vi "runServer.vi"(8 "error in (no error)":errorcluster, 11 "TcpServer in":refnum<class "TcpServer.lvclass">) -> (0 "error out (no error)":errorcluster, 3 "TcpServer out":refnum<class "TcpServer.lvclass">)   [LabVIEW 2018, in "TcpServer.lvclass"]
doc: "Run the TCP Server."
uses:
  TcpServer.lvclass
  TcpServer.lvclass/TcpServer.ctl
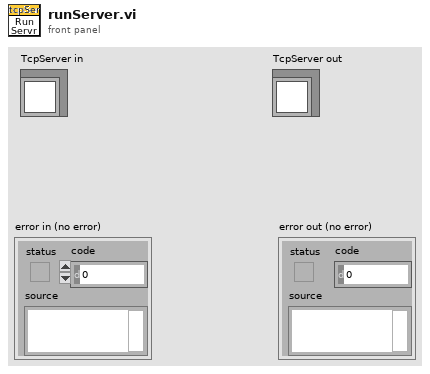
[diagram p1: front panel]
types:
  T1 = typedef "TcpServer.lvclass/userEventsTypeDef.ctl" = cluster{"TcpServer":refnum<user-event>, "Cmd":refnum<user-event>, "CmdStatus":refnum<user-event>, "Event":refnum<user-event>}
  T2 = enum16{"Standard", "Buffered", "CRLF", "Immediate"}
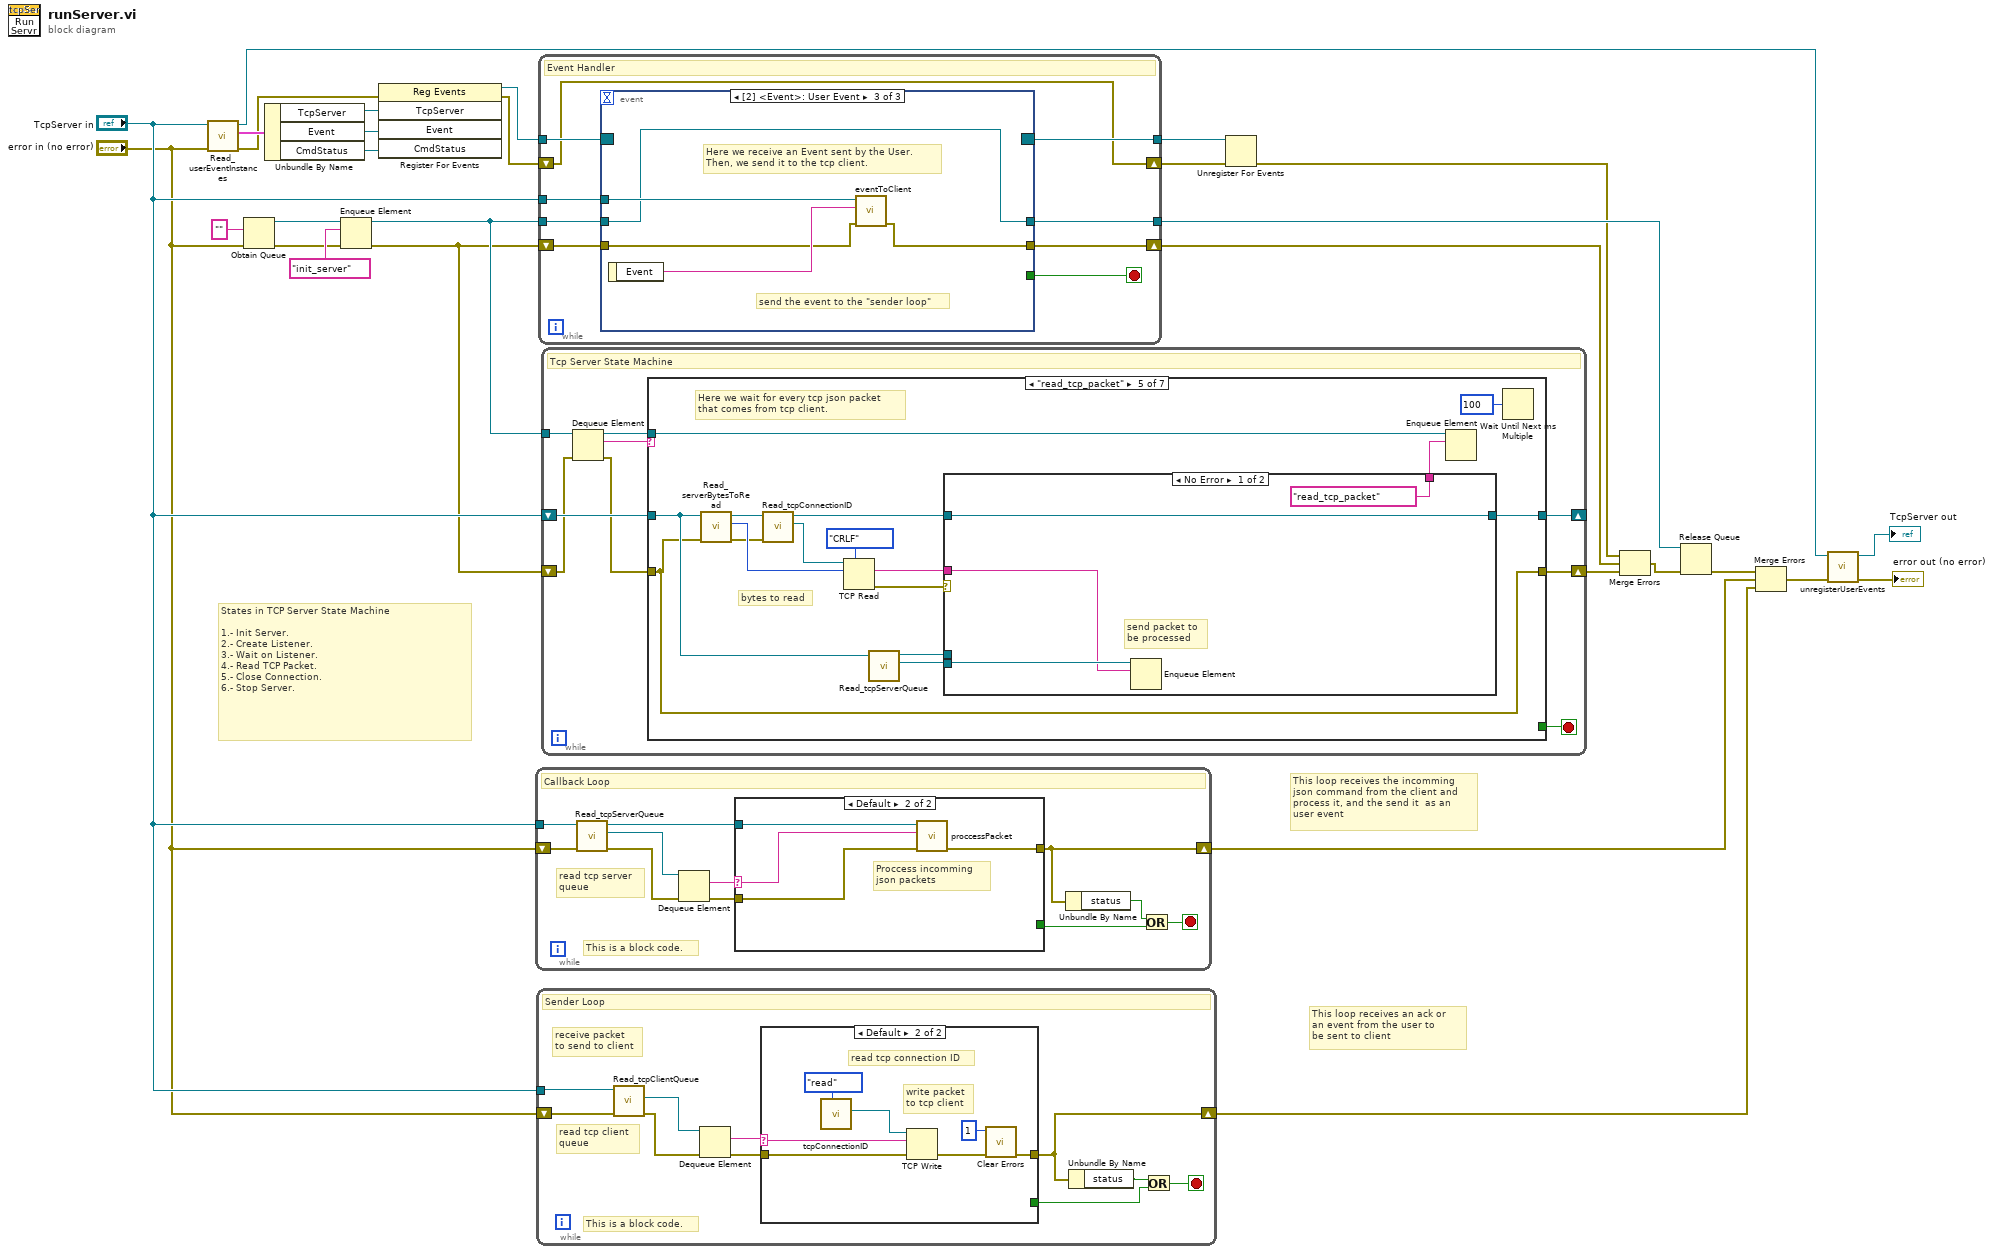
[diagram p0: block diagram]
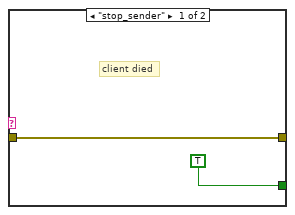
[diagram p2: hidden frame]
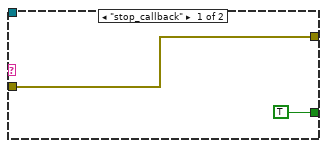
[diagram p3: hidden frame]
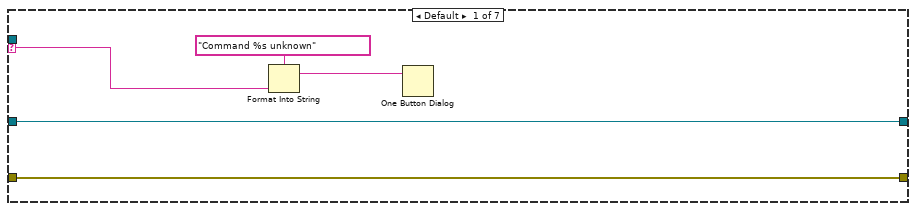
[diagram p4: hidden frame]
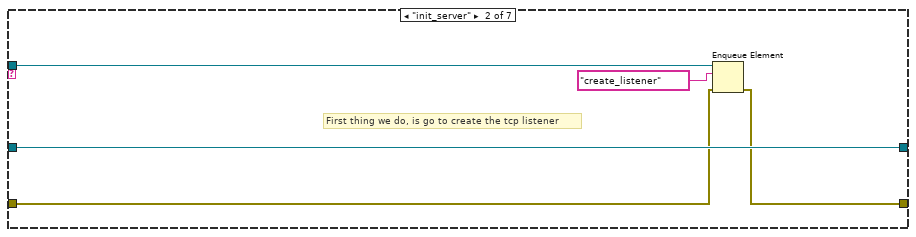
[diagram p5: hidden frame]
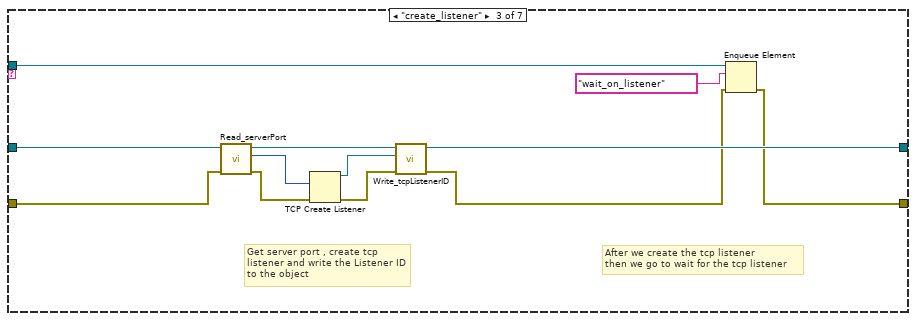
[diagram p6: hidden frame]
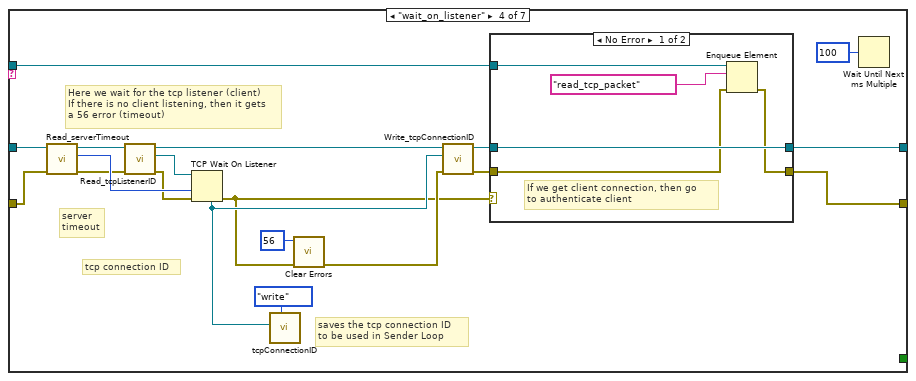
[diagram p7: hidden frame]
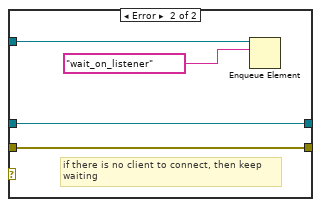
[diagram p8: hidden frame]
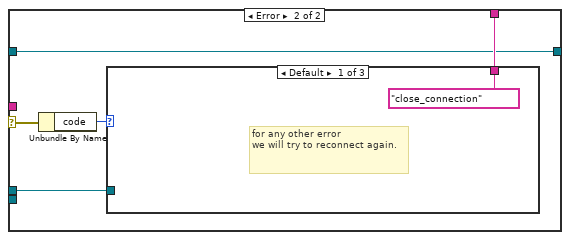
[diagram p9: hidden frame]
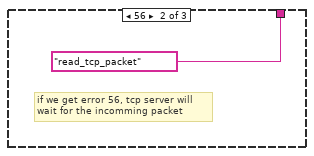
[diagram p10: hidden frame]
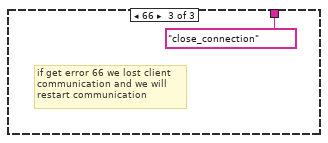
[diagram p11: hidden frame]
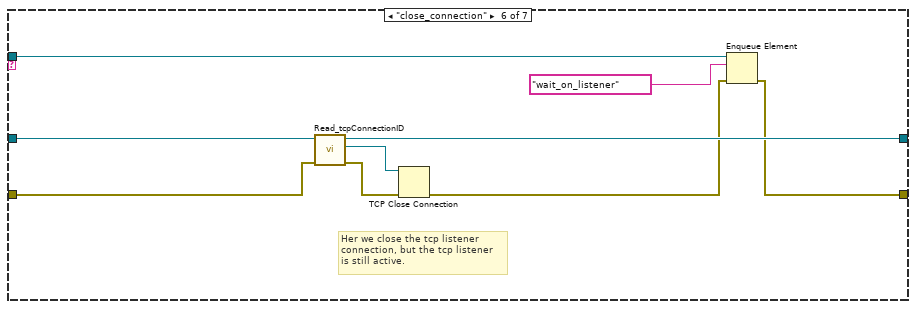
[diagram p12: hidden frame]
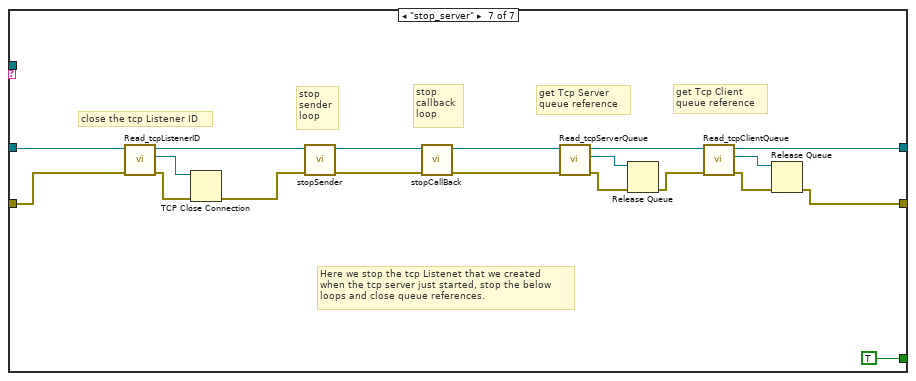
[diagram p13: hidden frame]
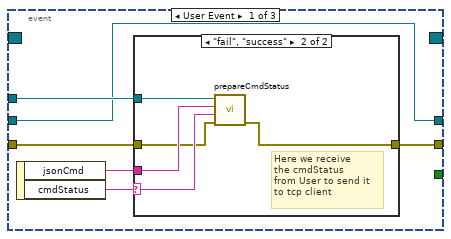
[diagram p14: hidden frame]
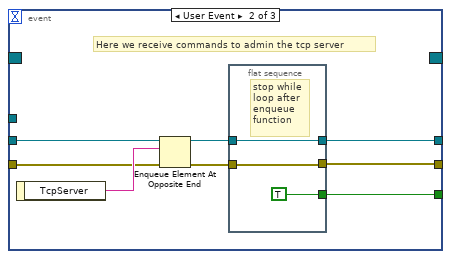
[diagram p16: hidden frame]
diagram:
  # "States in TCP Server State Machine\n\n1.- Init Server.\n2.- Create Listener.\n3.- Wait on Listener.\n4.- Read TCP Packet.\n5.- Close Connection.\n6.- Stop Server."
  # "This loop receives an ack or\nan event from the user to\nbe sent to client"
  # "This loop receives the incomming\njson command from the client and\nprocess it, and the send it  as an \nuser event"
  n1 = call "Read_userEventInstances.vi"("error in (no error)"="error in (no error)", "tcpServer in"="TcpServer in") -> ("error out"=w6:errorcluster, "UserEvents"=w27:T1, "tcpServer out"=w10:refnum<class "TcpServer.lvclass">)  [unwired: 7 in]
  n2 = Obtain Queue(element data type="", error in (no error)="error in (no error)") -> (queue out=w28:refnum<queue>, error out=w12:errorcluster)  [unwired: 3 in, 1 out]
  n3 = Unbundle By Name(w27) -> ("TcpServer"=w26:refnum<user-event>, "Event"=w21:refnum<user-event>, "CmdStatus"=w16:refnum<user-event>)
  n4 = Enqueue Element(queue=w28, element="init_server", error in (no error)=w12) -> (queue out=w24:refnum<queue>, error out=w7:errorcluster)  [unwired: 1 in, 1 out]
  n5 = register-events(error in=w6, w26, w21, w16) -> (reference out=w25:refnum<event-registration>, error out=w5:errorcluster)  [unwired: 1 in]
  n6 = while {
    tunnel: "TcpServer in" -> [w37]
    shift-right: [w31] -> w14
    shift-left: "error in (no error)" -> [w36]
    stop <- w33 stop-if-true
    # "This is a block code."
    # "read tcp server \nqueue"
    # "Callback Loop"
    n7 = call "Read_tcpServerQueue.vi"("error in (no error)"=w36, "tcpServer in"=w37) -> ("error out"=w35:errorcluster, "tcpServer queue"=w40:refnum<queue>, "tcpServer out"=w39:refnum<class "TcpServer.lvclass">)  [unwired: 7 in]
    n8 = Dequeue Element(queue=w40, error in (no error)=w35) -> (element=w38:string, error out=w34:errorcluster)  [unwired: 1 in, 2 out]
    n9 = case shown="Default" w38 {
      selector: w38 -> [_ w45]
      tunnel: w39 -> [_ w46]
      tunnel: [TRUE _] -> w32
      tunnel: w34 -> [w41 w44]
      tunnel: [w41 w43] -> w31
      frame "stop_callback" {
      }
      frame Default {
        # "Proccess incomming\njson packets"
        n10 = call "proccessPacket.vi"("error in (no error)"=w44, "tcp packet"=w45, "tcpServer in"=w46) -> ("error out"=w43:errorcluster)  [unwired: 7 in, 1 out]
      }
    }
    n11 = Unbundle By Name(w31) -> ("status"=w30:bool)
    n12 = Or(x=w30, y=w32) -> (x .or. y?=w33:bool)
  }
  n13 = while {
    tunnel: "TcpServer in" -> [w56]
    shift-right: [w47] -> w13
    shift-left: "error in (no error)" -> [w53]
    stop <- w52 stop-if-true
    # "This is a block code."
    # "receive packet\nto send to client"
    # "read tcp client \nqueue"
    # "Sender Loop"
    n14 = call "Read_tcpClientQueue.vi"("error in (no error)"=w53, "tcpServer in"=w56) -> ("error out"=w50:errorcluster, "tcpClient queue"=w54:refnum<queue>)  [unwired: 7 in, 1 out]
    n15 = Dequeue Element(queue=w54, error in (no error)=w50) -> (element=w55:string, error out=w49:errorcluster)  [unwired: 1 in, 2 out]
    n16 = case shown="Default" w55 {
      selector: w55 -> [_ w65]
      tunnel: [TRUE _] -> w51
      tunnel: w49 -> [w57 w59]
      tunnel: [w57 w60] -> w47
      frame "stop_sender" {
        # "client died"
      }
      frame Default {
        # "write packet\nto tcp client"
        # "read tcp connection ID"
        n17 = call "tcpConnectionID.vi"("function"=enum16{"read", "write"}."read") -> ("connection ID out"=w63:refnum<k5>)  [unwired: 10 in]
        n18 = TCP Write(connection ID=w63, data in=w65, error in (no error)=w59) -> (error out=w61:errorcluster)  [unwired: 1 in, 2 out]
        n19 = call <vilib>:"Clear Errors.vi"("error in (no error)"=w61, "specific error code to clear (0: all)"=1) -> ("error out"=w60:errorcluster)  [unwired: 4 in, 1 out]
      }
    }
    n20 = Unbundle By Name(w47) -> ("status"=w48:bool)
    n21 = Or(x=w48, y=w51) -> (x .or. y?=w52:bool)
  }
  n22 = while {
    tunnel: w24 -> [w74]
    tunnel: w25 -> [w73]
    tunnel: [w71] -> w22
    tunnel: "TcpServer in" -> [w70]
    tunnel: [w69] -> w8
    shift-right: [w66] -> w3
    shift-left: w5 -> [w66]
    shift-right: [w67] -> w1
    shift-left: w7 -> [w68]
    stop <- w72 stop-if-true
    # "Event Handler"
    n23 = event shown="[2] <Event>: User Event" {
      selector: w73 -> [_ _ _]
      dyn-events: [_ _ _] -> w69
      timeout: _ -> [_ _ _]
      tunnel: w74 -> [w75 w94 w100]
      tunnel: [_ w92 _] -> w72
      tunnel: [w75 w90 w100] -> w71
      tunnel: w70 -> [w78 _ w102]
      tunnel: w68 -> [w77 w89 w99]
      tunnel: [w76 w87 w98] -> w67
      event User Event {
        n24 = event-data() -> ("jsonCmd"=w79:string, "cmdStatus"=w80:string)  [unwired: 1 in]
        n25 = case shown="\"fail\", \"success\"" w80 {
          selector: w80 -> [_ w84]
          tunnel: w79 -> [_ w85]
          tunnel: w78 -> [_ w86]
          tunnel: w77 -> [w81 w83]
          tunnel: [w81 w82] -> w76
          frame Default {
          }
          frame "fail", "success" {
            # "Here we receive \nthe cmdStatus\nfrom User to send it \nto tcp client"
            n26 = call "prepareCmdStatus.vi"("error in (no error)"=w83, "cmdStatus"=w84, "cmd"=w85, "tcpServer in"=w86) -> ("error out"=w82:errorcluster)  [unwired: 6 in, 1 out]
          }
        }
      }
      event User Event {
        # "Here we receive commands to admin the tcp server"
        n27 = event-data() -> ("TcpServer"=w93:string)  [unwired: 1 in]
        n28 = Enqueue Element At Opposite End(queue=w94, element=w93, error in (no error)=w89) -> (queue out=w91:refnum<queue>, error out=w88:errorcluster)  [unwired: 1 in, 1 out]
        n29 = flat-sequence {
          tunnel: [TRUE] -> w92
          tunnel: w91 -> [w96]
          tunnel: [w96] -> w90
          tunnel: w88 -> [w95]
          tunnel: [w95] -> w87
          frame #0 {
            # "stop while\nloop after\nenqueue\nfunction"
          }
        }
      }
      event User Event {
        # "Here we receive an Event sent by the User.\nThen, we send it to the tcp client."
        # "send the event to the \"sender loop\""
        n30 = event-data() -> ("Event"=w101:string)  [unwired: 1 in]
        n31 = call "eventToClient.vi"("error in (no error)"=w99, "evtName"=w101, "TcpServer in"=w102) -> ("error out"=w98:errorcluster)  [unwired: 7 in, 1 out]
      }
    }
  }
  n32 = while {
    tunnel: w24 -> [w111]
    shift-right: [w109] -> _
    shift-left: "TcpServer in" -> [w110]
    shift-right: [w105] -> w19
    shift-left: w7 -> [w104]
    stop <- w106 stop-if-true
    # "Tcp Server State Machine"
    n33 = Dequeue Element(queue=w111, error in (no error)=w104) -> (queue out=w108:refnum<queue>, element=w107:string, error out=w103:errorcluster)  [unwired: 1 in, 1 out]
    n34 = case shown="\"read_tcp_packet\"" w107 {
      selector: w107 -> [w115 _ _ _ _ _ _]
      tunnel: w110 -> [w113 w121 w131 w149 w172 w198 w216]
      tunnel: [w113 w121 w127 w148 w167 w195 w211] -> w109
      tunnel: w108 -> [_ w120 w126 w147 w170 w197 _]
      tunnel: [_ _ _ _ _ _ TRUE] -> w106
      tunnel: w103 -> [w112 w118 w124 w142 w164 w193 w207]
      tunnel: [w112 w117 w122 w135 w164 w190 w199] -> w105
      frame Default {
        n35 = Format Into String(format string="Command %s unknown", w115) -> (resulting string=w114:string)  [unwired: 2 in, 1 out]
        n36 = One Button Dialog(message=w114) -> ()  [unwired: 1 in, 1 out]
      }
      frame "init_server" {
        # "First thing we do, is go to create the tcp listener"
        n37 = Enqueue Element(queue=w120, element="create_listener", error in (no error)=w118) -> (error out=w117:errorcluster)  [unwired: 1 in, 2 out]
      }
      frame "create_listener" {
        # "After we create the tcp listener\nthen we go to wait for the tcp listener"
        # "Get server port , create tcp listener and write the Listener ID to the object"
        n38 = call "Read_serverPort.vi"("error in (no error)"=w124, "tcpServer in"=w131) -> ("error out"=w132:errorcluster, "serverPort"=w133:u16, "tcpServer out"=w130:refnum<class "TcpServer.lvclass">)  [unwired: 7 in]
        n39 = TCP Create Listener(8:w132, 10:w133) -> (0:w128:errorcluster, 3:w129:refnum<k5>)  [unwired: 3 in, 1 out]
        n40 = call "Write_tcpListenerID.vi"("error in (no error)"=w128, "tcpListenerID"=w129, "tcpServer in"=w130) -> ("error out"=w123:errorcluster, "tcpServer out"=w127:refnum<class "TcpServer.lvclass">)  [unwired: 7 in]
        n41 = Enqueue Element(queue=w126, element="wait_on_listener", error in (no error)=w123) -> (error out=w122:errorcluster)  [unwired: 1 in, 2 out]
      }
      frame "wait_on_listener" {
        # "Here we wait for the tcp listener (client)\nIf there is no client listening, then it gets\na 56 error (timeout)"
        # "tcp connection ID"
        # "saves the tcp connection ID\nto be used in Sender Loop"
        # "server\ntimeout"
        n42 = call "Read_serverTimeout.vi"("error in (no error)"=w142, "tcpServer in"=w149) -> ("error out"=w141:errorcluster, "serverTimeout"=w150:i32, "tcpServer out"=w151:refnum<class "TcpServer.lvclass">)  [unwired: 7 in]
        n43 = call "Read_tcpListenerID.vi"("error in (no error)"=w141, "tcpServer in"=w151) -> ("error out"=w140:errorcluster, "tcpListenerID"=w152:refnum<k5>, "tcpServer out"=w146:refnum<class "TcpServer.lvclass">)  [unwired: 7 in]
        n44 = TCP Wait On Listener(8:w140, 9:w150, 11:w152) -> (0:w137:errorcluster, 4:w143:refnum<k5>)  [unwired: 1 in, 3 out]
        n45 = call "tcpConnectionID.vi"("function"=enum16{"read", "write"}."write", "connection ID"=w143) -> ()  [unwired: 9 in, 1 out]
        n46 = call <vilib>:"Clear Errors.vi"("error in (no error)"=w137, "specific error code to clear (0: all)"=56) -> ("error out"=w138:errorcluster)  [unwired: 4 in, 1 out]
        n47 = call "Write_tcpConnectionID.vi"("error in (no error)"=w138, "tcpConnectionID"=w143, "TcpServer in"=w146) -> ("error out"=w136:errorcluster, "TcpServer out"=w145:refnum<class "TcpServer.lvclass">)  [unwired: 7 in]
        n48 = case shown="No Error" w137 {
          tunnel: w145 -> [w157 w161]
          tunnel: [w157 w161] -> w148
          tunnel: w147 -> [w155 w160]
          tunnel: w136 -> [w154 w158]
          tunnel: [w153 w158] -> w135
          frame No Error {
            # "If we get client connection, then go \nto authenticate client"
            n49 = Enqueue Element(queue=w155, element="read_tcp_packet", error in (no error)=w154) -> (error out=w153:errorcluster)  [unwired: 1 in, 2 out]
          }
          frame Error {
            # "if there is no client to connect, then keep\nwaiting"
            n50 = Enqueue Element(queue=w160, element="wait_on_listener") -> ()  [unwired: 2 in, 3 out]
          }
        }
        n51 = Wait Until Next ms Multiple(millisecond multiple=u32 100) -> ()  [unwired: 1 out]
      }
      frame "read_tcp_packet" {
        # "Here we wait for every tcp json packet\nthat comes from tcp client."
        # "bytes to read"
        n52 = call "Read_serverBytesToRead.vi"("error in (no error)"=w164, "tcpServer in"=w172) -> ("error out"=w165:errorcluster, "serverBytesToRead"=w174:i32, "tcpServer out"=w171:refnum<class "TcpServer.lvclass">)  [unwired: 7 in]
        n53 = call "Read_tcpConnectionID.vi"("error in (no error)"=w165, "TcpServer in"=w171) -> ("tcpConnectionID"=w166:refnum<k5>, "TcpServer out"=w168:refnum<class "TcpServer.lvclass">)  [unwired: 7 in, 1 out]
        n54 = TCP Read(connection ID=w166, bytes to read=w174, 7:T2."CRLF" ("mode (standard)")) -> (data out=w177:string, error out=w175:errorcluster)  [unwired: 2 in, 1 out]
        n55 = call "Read_tcpServerQueue.vi"("tcpServer in"=w172) -> ("tcpServer queue"=w163:refnum<queue>, "tcpServer out"=w173:refnum<class "TcpServer.lvclass">)  [unwired: 8 in, 1 out]
        n56 = case shown="No Error" w175 {
          selector: w175 -> [_ w186]
          tunnel: w177 -> [w178 _]
          tunnel: w163 -> [w181 _]
          tunnel: w173 -> [_ w184]
          tunnel: ["read_tcp_packet" w183] -> w169
          tunnel: w168 -> [w179 w182]
          tunnel: [w179 w182] -> w167
          frame No Error {
            # "send packet to\nbe processed"
            n57 = Enqueue Element(queue=w181, element=w178) -> ()  [unwired: 2 in, 3 out]
          }
          frame Error {
            n58 = Unbundle By Name(w186) -> ("code"=w185:i32)
            n59 = case shown="Default" w185 {
              tunnel: w184 -> [_ _ _]
              tunnel: ["close_connection" "read_tcp_packet" "close_connection"] -> w183
              frame Default {
                # "for any other error\nwe will try to reconnect again."
              }
              frame 56 {
                # "if we get error 56, tcp server will \nwait for the incomming packet"
              }
              frame 66 {
                # "if get error 66 we lost client \ncommunication and we will\nrestart communication"
              }
            }
          }
        }
        n60 = Enqueue Element(queue=w170, element=w169) -> ()  [unwired: 2 in, 3 out]
        n61 = Wait Until Next ms Multiple(millisecond multiple=u32 100) -> ()  [unwired: 1 out]
      }
      frame "close_connection" {
        # "Her we close the tcp listener\nconnection, but the tcp listener\nis still active."
        n62 = call "Read_tcpConnectionID.vi"("error in (no error)"=w193, "TcpServer in"=w198) -> ("error out"=w192:errorcluster, "tcpConnectionID"=w194:refnum<k5>, "TcpServer out"=w195:refnum<class "TcpServer.lvclass">)  [unwired: 7 in]
        n63 = TCP Close Connection(connection ID=w194, error in (no error)=w192) -> (error out=w191:errorcluster)  [unwired: 1 in, 1 out]
        n64 = Enqueue Element(queue=w197, element="wait_on_listener", error in (no error)=w191) -> (error out=w190:errorcluster)  [unwired: 1 in, 2 out]
      }
      frame "stop_server" {
        # "Here we stop the tcp Listenet that we created\nwhen the tcp server just started, stop the below\nloops and close queue references."
        # "close the tcp Listener ID"
        # "stop\nsender\nloop"
        # "stop\ncallback\nloop"
        # "get Tcp Client \nqueue reference"
        # "get Tcp Server \nqueue reference"
        n65 = call "Read_tcpListenerID.vi"("error in (no error)"=w207, "tcpServer in"=w216) -> ("error out"=w206:errorcluster, "tcpListenerID"=w217:refnum<k5>, "tcpServer out"=w209:refnum<class "TcpServer.lvclass">)  [unwired: 7 in]
        n66 = TCP Close Connection(connection ID=w217, error in (no error)=w206) -> (error out=w205:errorcluster)  [unwired: 1 in, 1 out]
        n67 = call "stopSender.vi"("error in (no error)"=w205, "TcpServer in"=w209) -> ("error out"=w204:errorcluster, "TcpServer out"=w210:refnum<class "TcpServer.lvclass">)  [unwired: 8 in]
        n68 = call "stopCallBack.vi"("error in (no error)"=w204, "TcpServer in"=w210) -> ("error out"=w203:errorcluster, "TcpServer out"=w208:refnum<class "TcpServer.lvclass">)  [unwired: 8 in]
        n69 = call "Read_tcpServerQueue.vi"("error in (no error)"=w203, "tcpServer in"=w208) -> ("error out"=w202:errorcluster, "tcpServer queue"=w214:refnum<queue>, "tcpServer out"=w213:refnum<class "TcpServer.lvclass">)  [unwired: 7 in]
        n70 = Release Queue(queue=w214, error in (no error)=w202) -> (error out=w201:errorcluster)  [unwired: 1 in, 2 out]
        n71 = call "Read_tcpClientQueue.vi"("error in (no error)"=w201, "tcpServer in"=w213) -> ("error out"=w200:errorcluster, "tcpClient queue"=w212:refnum<queue>, "tcpServer out"=w211:refnum<class "TcpServer.lvclass">)  [unwired: 7 in]
        n72 = Release Queue(queue=w212, error in (no error)=w200) -> (error out=w199:errorcluster)  [unwired: 1 in, 2 out]
      }
    }
  }
  n73 = Unregister For Events(event registration refnum=w8, error in=w3) -> (error out=w2:errorcluster)
  n74 = Merge Errors(w2, w1, w19) -> (w4:errorcluster)
  n75 = Release Queue(queue=w22, error in (no error)=w4) -> (error out=w17:errorcluster)  [unwired: 1 in, 2 out]
  n76 = Merge Errors(w17, w14, w13) -> (w15:errorcluster)
  n77 = call "unregisterUserEvents.vi"("error in (no error)"=w15, "tcpServer in"=w10) -> ("error out"=→"error out (no error)":errorcluster, "tcpServer out"=→"TcpServer out":refnum<class "TcpServer.lvclass">)  [unwired: 8 in]
